vi "Enqueue Blocking Callbacks.vi"(8 "error in (no error)":errorcluster, 10 "Array":refnum<class "Blocking Callback.lvclass">[](array[class]), 11 "Future in":refnum<class "Future.lvclass">) -> (0 "error out":errorcluster, 3 "Future out":refnum<class "Future.lvclass">)   [LabVIEW 2017, in "Promise Future.lvlib" / "Future.lvclass"]
uses:
  Future.lvclass
  Callback/Blocking Callback.lvclass
  E:/Promise/Promise Future/Callback/Callback.lvclass
  Future.lvclass/Future.ctl
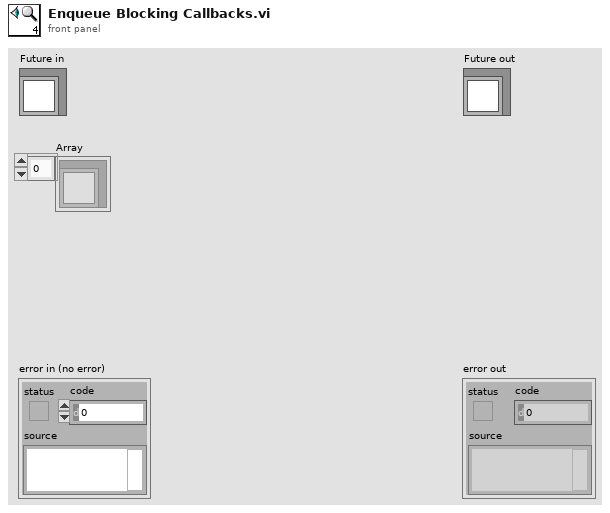
[diagram p1: front panel]
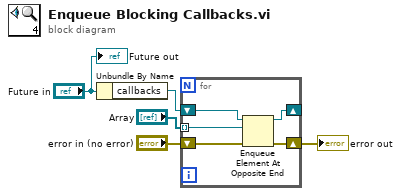
[diagram p0: block diagram]
diagram:
  n1 = Unbundle By Name("Future in") -> ("callbacks"=w2:refnum<queue>)
  n2 = for {
    shift-right: [w6] -> w4
    shift-left: "error in (no error)" -> [w8]
    shift-right: [w7] -> _
    shift-left: w2 -> [w10]
    tunnel: "Array" -> [w9] mode=indexing
    n3 = Enqueue Element At Opposite End(queue=w10, element=w9, error in (no error)=w8) -> (queue out=w7:refnum<queue>, error out=w6:errorcluster)  [unwired: 1 in, 1 out]
  }
  "error out" <- w4
  "Future out" <- "Future in"
